vi "Graficas.vi"(1 "ID_EQUIPO":i32=1, 2 "Generador in":string) -> ()   [LabVIEW 2018]
uses:
  <vilib>/RAFA Solutions/Harmony UI Controls Kit/String & Path/String Indicator.ctl
  <vilib>/RAFA Solutions/Harmony UI Controls Kit/Boolean/OK Button.ctl
  <vilib>/addons/Electrical Power/Basic/Controls/Vector Diagram/EPX Vector Diagram.xctl
  Controls/Cluster_Potencias.ctl
  <vilib>/RAFA Solutions/Harmony UI Controls Kit/Numeric/Horizontal Progress Bar.ctl
  <vilib>/RAFA Solutions/Harmony UI Controls Kit/Boolean/Radio Button.ctl
  <vilib>/RAFA Solutions/Harmony UI Controls Kit/Boolean/Round Led.ctl
  Controls/Hora y Fecha control.ctl
  <vilib>/RAFA Solutions/Harmony UI Controls Kit/Boolean/Blank Button - Blue.ctl
  <vilib>/addons/database/Connection.llb/DB Tools Open Connec (Path).vi
  Global/Demo.vi
  Global/globalEventos.vi
  Global/Alarmas_indicadores-LED.vi
  <vilib>/RAFA Solutions/Harmony UI Controls Kit/Flat UI Design.lvlib
  <vilib>/addons/database/NI_Database_API.lvlib
panel:
  in  "type specifier VI Refnum (for type only) 2":refnum<vi>
  in  "ok":T1
  out "fecha y hora":T2
  out "Tol_Frec":T3 caption="TOL: Frecuencia"
  out "Mod_Frec":T3 caption="MOD: Frecuencia"
  out "Tol_V3_V1":T3 caption="TOL: V3_V1"
  out "Tol_V2_V3":T3 caption="TOL: V2_V3"
  out "Tol_V1_V2":T3 caption="TOL: V1_V2"
  out "Mod_V3_V1":T3 caption="MOD: V3_V1"
  out "Mod_V2_V3":T3 caption="MOD: V2_V3"
  out "Mod_V1_V2":T3 caption="MOD: V1_V2"
  out "G1_TRANS":T3 caption="Transiente"
  out "G1_SWELL":T3 caption="Swell"
  out "G1_SAG":T3 caption="Sag"
  in  "Seleccion Armonicos":T4(radio)
  out "Armónicos":sgl[](graph)
  out "?":sgl format="%#_3f"
  out "?":sgl format="%#_2f"
  out "?":sgl format="%#.1f"
  out "PROM":T5 scale=0.0..100.0
  out "L3-L1":T5 scale=0.0..100.0
  out "L2-L3":T5 scale=0.0..100.0
  out "L1-L2":T5 scale=0.0..100.0
  out "PROM.":T5 scale=0.0..100.0
  out "L3-L1":T5 scale=0.0..100.0
  out "L2-L3":T5 scale=0.0..100.0
  out "L1-L2":T5 scale=0.0..100.0
  out "TOTAL":T6 {"FACT. POT." scale=0.0..1.0; "APARENTE" scale=0.0..500.0; "REACTIVA" scale=0.0..500.0; "ACTIVA" scale=0.0..700.0}
  out "V3_V1":T6 {"FACT. POT." scale=0.0..1.0; "APARENTE" scale=0.0..500.0; "REACTIVA" scale=0.0..500.0; "ACTIVA" scale=0.0..700.0}
  out "V2-V3":T6 {"FACT. POT." scale=0.0..1.0; "APARENTE" scale=0.0..500.0; "REACTIVA" scale=0.0..500.0; "ACTIVA" scale=0.0..700.0}
  out "V1-V2":T6 {"FACT. POT." scale=0.0..1.0; "APARENTE" scale=0.0..500.0; "REACTIVA" scale=0.0..500.0; "ACTIVA" scale=0.0..700.0}
  out "Generador":string
  out "Corriente Vector Diagram":cdb[](xcontrol)
  out "Voltage Vector Diagram":cdb[](xcontrol)
  out "Frecuencia":cluster{"V1_V2":sgl, "V2_V3":sgl, "V3_V1":sgl}(graph)
  out "Corriente L_L":cluster{"V1_V2":sgl, "V2_V3":sgl, "V3_V1":sgl}(graph)
  out "Voltaje L-L":T7(graph)
  in  "volver":T8
  out "Eventos":T9
  # "Sistema de Monitoreo de Calidad de Energía"
  # "VOLTAJES L-L (RMS)"
  # "Gráfica Polar de Voltaje"
  # "POTENCIAS"
  # "VOLTAJE PROM."
  # "V"
  # "VALOR PROMEDIO \nV1-V2-V3"
  # "Límites de tolerancia según IEEE45"
  # "CORRIENTE PROM"
  # "A"
  # "VALOR PROMEDIO \nI1-I2-I3"
  # "CORRIENTES (RMS)"
  # "Gráfica Polar de Corriente"
  # "FRECUENCIA"
  # "Hz"
  # "THD VOLTAJE"
  # "THD CORRIENTE"
  # "%"
  # "%"
  # "ALARMAS"
  # "%"
  # "%"
  # "%"
  # "%"
  # "%"
  # "%"
  # "FRECUENCIA GENERADA"
  # "ARMÓNICOS"
  # "Límites de tolerancia según IEEE45"
  # "kW"
  # "kVAR"
  # "kVA"
  # "-"
  # "kW"
  # "kVAR"
  # "kVA"
  # "-"
  # "kW"
  # "kVAR"
  # "kVA"
  # "-"
  # "kW"
  # "kVAR"
  # "kVA"
  # "-"
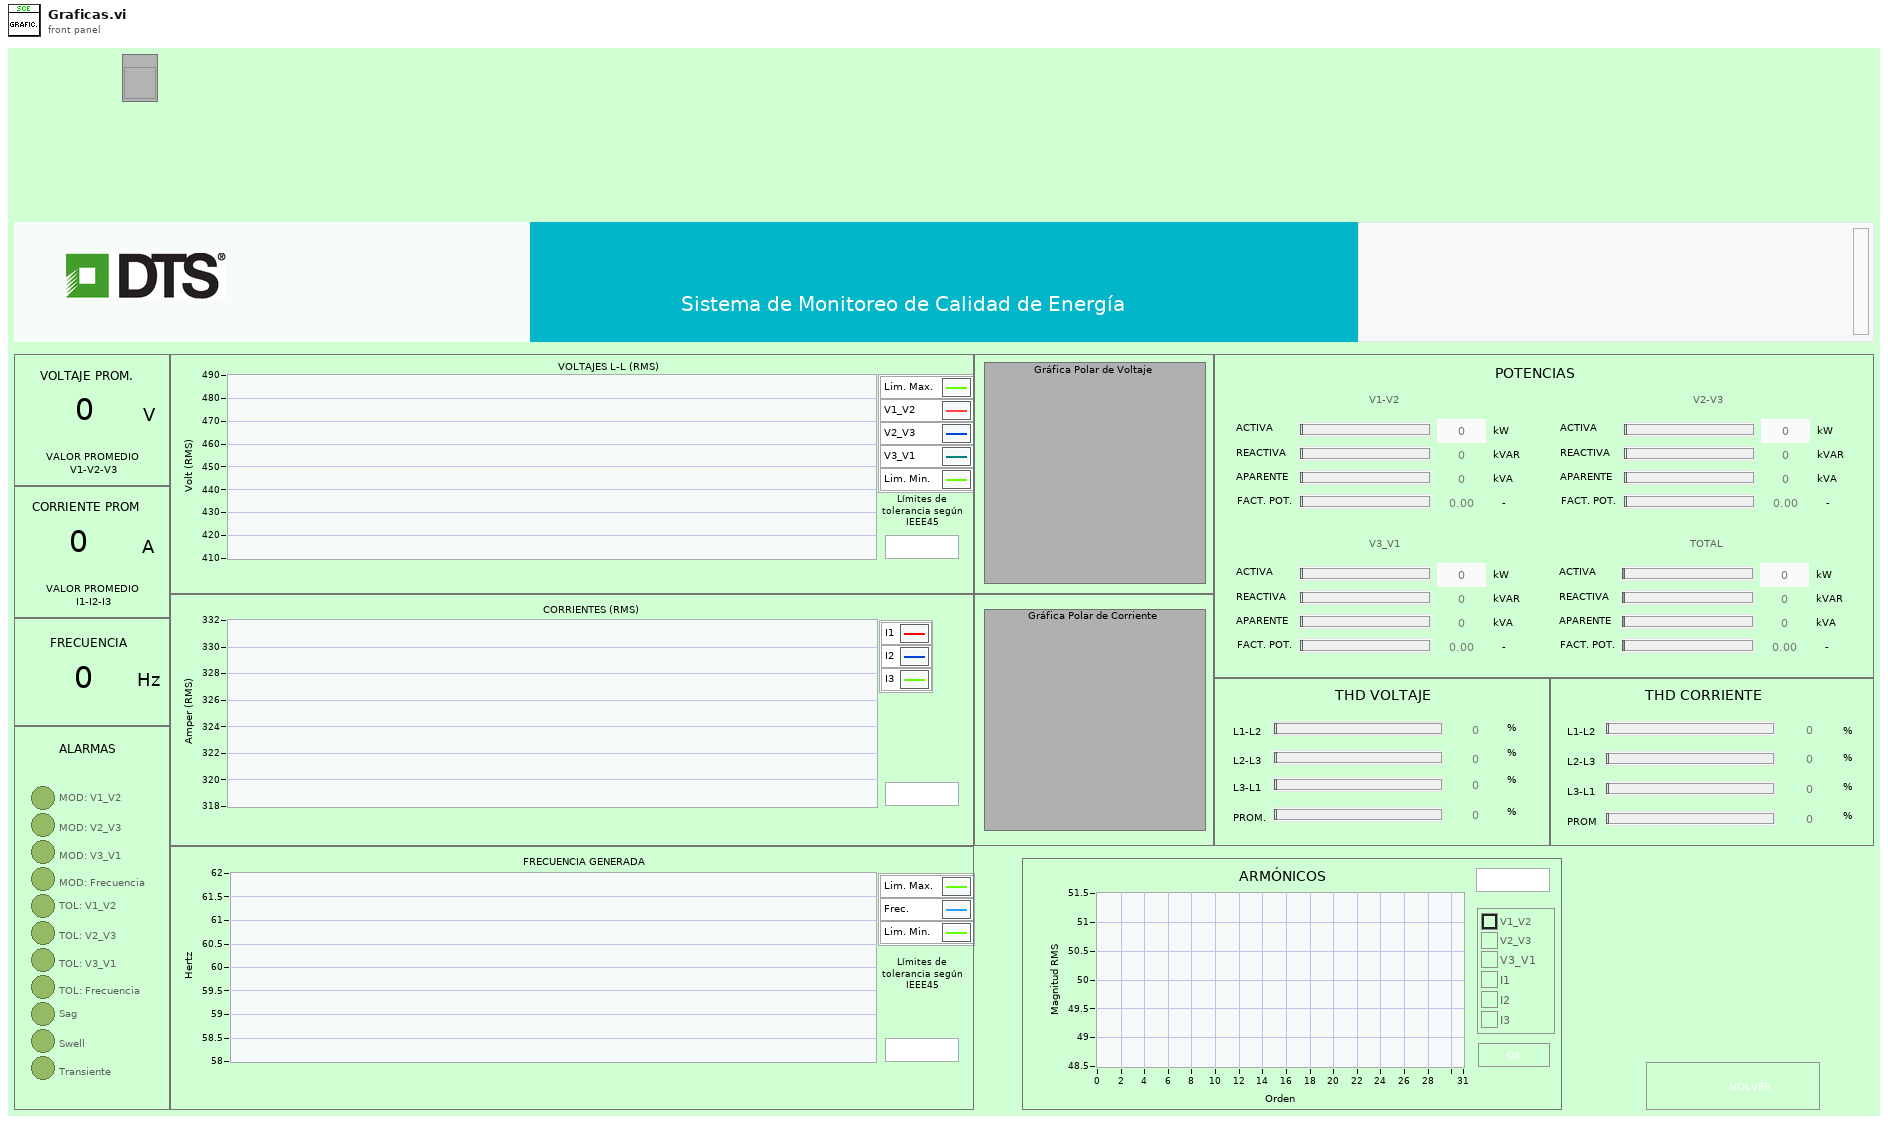
[diagram p1: front panel]
types:
  T1 = typedef "Flat UI Design.lvlib/Blank Button - Blue.ctl" = bool
  T2 = typedef "Hora y Fecha control.ctl" = cluster{"fecha":string, "dia semana":string, "fecha 2":string}
  T3 = typedef "Flat UI Design.lvlib/Round Led.ctl" = bool
  T4 = enum32{"V1_V2", "V2_V3", "V3_V1", "I1", "I2", "I3"}
  T5 = typedef "Flat UI Design.lvlib/Horizontal Progress Bar.ctl" = sgl
  T6 = typedef "Cluster_Potencias.ctl" = cluster{"ACTIVA":T5, "REACTIVA":T5, "APARENTE":T5, "FACT. POT.":T5}
  T7 = cluster{"Max":sgl, "V1_V2":sgl, "V2_V3":sgl, "V3_V1":sgl, "Min":sgl}
  T8 = typedef "Flat UI Design.lvlib/OK Button.ctl" = bool
  T9 = typedef "Flat UI Design.lvlib/String Indicator.ctl" = string
  T10 = cluster{"Max":sgl, "V1_V2":sgl, "V2_V3":sgl, "V3_V1":sgl, "Min":sgl}[]
  T11 = typedef "NI_Database_API.lvlib/Conn ObjectReference.ctl" = refnum<k1>
  T12 = cluster{"V_polar":cluster{"V1_ang":sgl, "V1_mag":sgl, "V2_ang":sgl, "V2_mag":sgl, "V3_ang":sgl, "V3_mag":sgl}, "I_polar":cluster{"I1_ang":sgl, "I1_mag":sgl, "I2_ang":sgl, "I2_mag":sgl, "I3_ang":sgl, "I3_mag":sgl}}
  T13 = typedef "THD_cluster.ctl" = cluster{"V_THD":cluster{"V1_V2_THD":sgl, "V2_V3_THD":sgl, "V3_V1_THD":sgl, "Avg_V_V_THD":sgl}, "I_THD":cluster{"I1_THD":sgl, "I2_THD":sgl, "I3_THD":sgl, "I4_THD":sgl, "Avg_I_THD":sgl}}
  T14 = cluster{"V1_V2_THD":sgl, "V2_V3_THD":sgl, "V3_V1_THD":sgl, "Avg_V_V_THD":sgl}
  T15 = cluster{"I1_THD":sgl, "I2_THD":sgl, "I3_THD":sgl, "I4_THD":sgl, "Avg_I_THD":sgl}
  T16 = cluster{"Real Power (kW)":cluster{"L1_kW":sgl, "L2_kW":sgl, "L3_kW":sgl, "Total_kW":sgl}, "Reactive Power (kVAR)":cluster{"L1_kVAR":sgl, "L2_kVAR":sgl, "L3_kVAR":sgl, "Total_kVAR":sgl}, "Aparent Power (kVA)":cluster{"L1_kVA":sgl, "L2_kVA":sgl, "L3_kVA":sgl, "Total_kVA":sgl}, "Power Factor":cluster{"L1_PF":sgl, "L2_PF":sgl, "L3_PF":sgl, "Total_PF":sgl}}
  T17 = cluster{"Real Power (kW)":cluster{"L1_kW":sgl, "L2_kW":sgl, "L3_kW":sgl, "Total_kW":sgl}, "Reactive Power (kVAR)":cluster{"L1_kVAR":sgl, "L2_kVAR":sgl, "L3_kVAR":sgl, "Total_kVAR":sgl}, "Aparent Power (kVA)":cluster{"L1_kVA":sgl, "L2_kVA":sgl, "L3_kVA":sgl, "Total_kVA":sgl}, "Power Factor (%)":cluster{"L1_PF":sgl, "L2_PF":sgl, "L3_PF":sgl, "Total_PF":sgl}}
  T18 = cluster{"L1_kW":sgl, "L2_kW":sgl, "L3_kW":sgl, "Total_kW":sgl}
  T19 = cluster{"L1_kVAR":sgl, "L2_kVAR":sgl, "L3_kVAR":sgl, "Total_kVAR":sgl}
  T20 = cluster{"L1_kVA":sgl, "L2_kVA":sgl, "L3_kVA":sgl, "Total_kVA":sgl}
  T21 = cluster{"L1_PF":sgl, "L2_PF":sgl, "L3_PF":sgl, "Total_PF":sgl}
  T22 = typedef "VIF_cluster.ctl" = cluster{"VL_VL":cluster{"V1_V2":sgl, "V2_V3":sgl, "V3_V1":sgl, "Avg_VL_VL":sgl}, "IL_IL":cluster{"I1":sgl, "I2":sgl, "I3":sgl, "Avg_Amps":sgl}, "Frecuency":sgl, "Avg_Frecuency":sgl}
  T23 = cluster{"V1_V2":sgl, "V2_V3":sgl, "V3_V1":sgl, "Avg_VL_VL":sgl}
  T24 = cluster{"I1":sgl, "I2":sgl, "I3":sgl, "Avg_Amps":sgl}
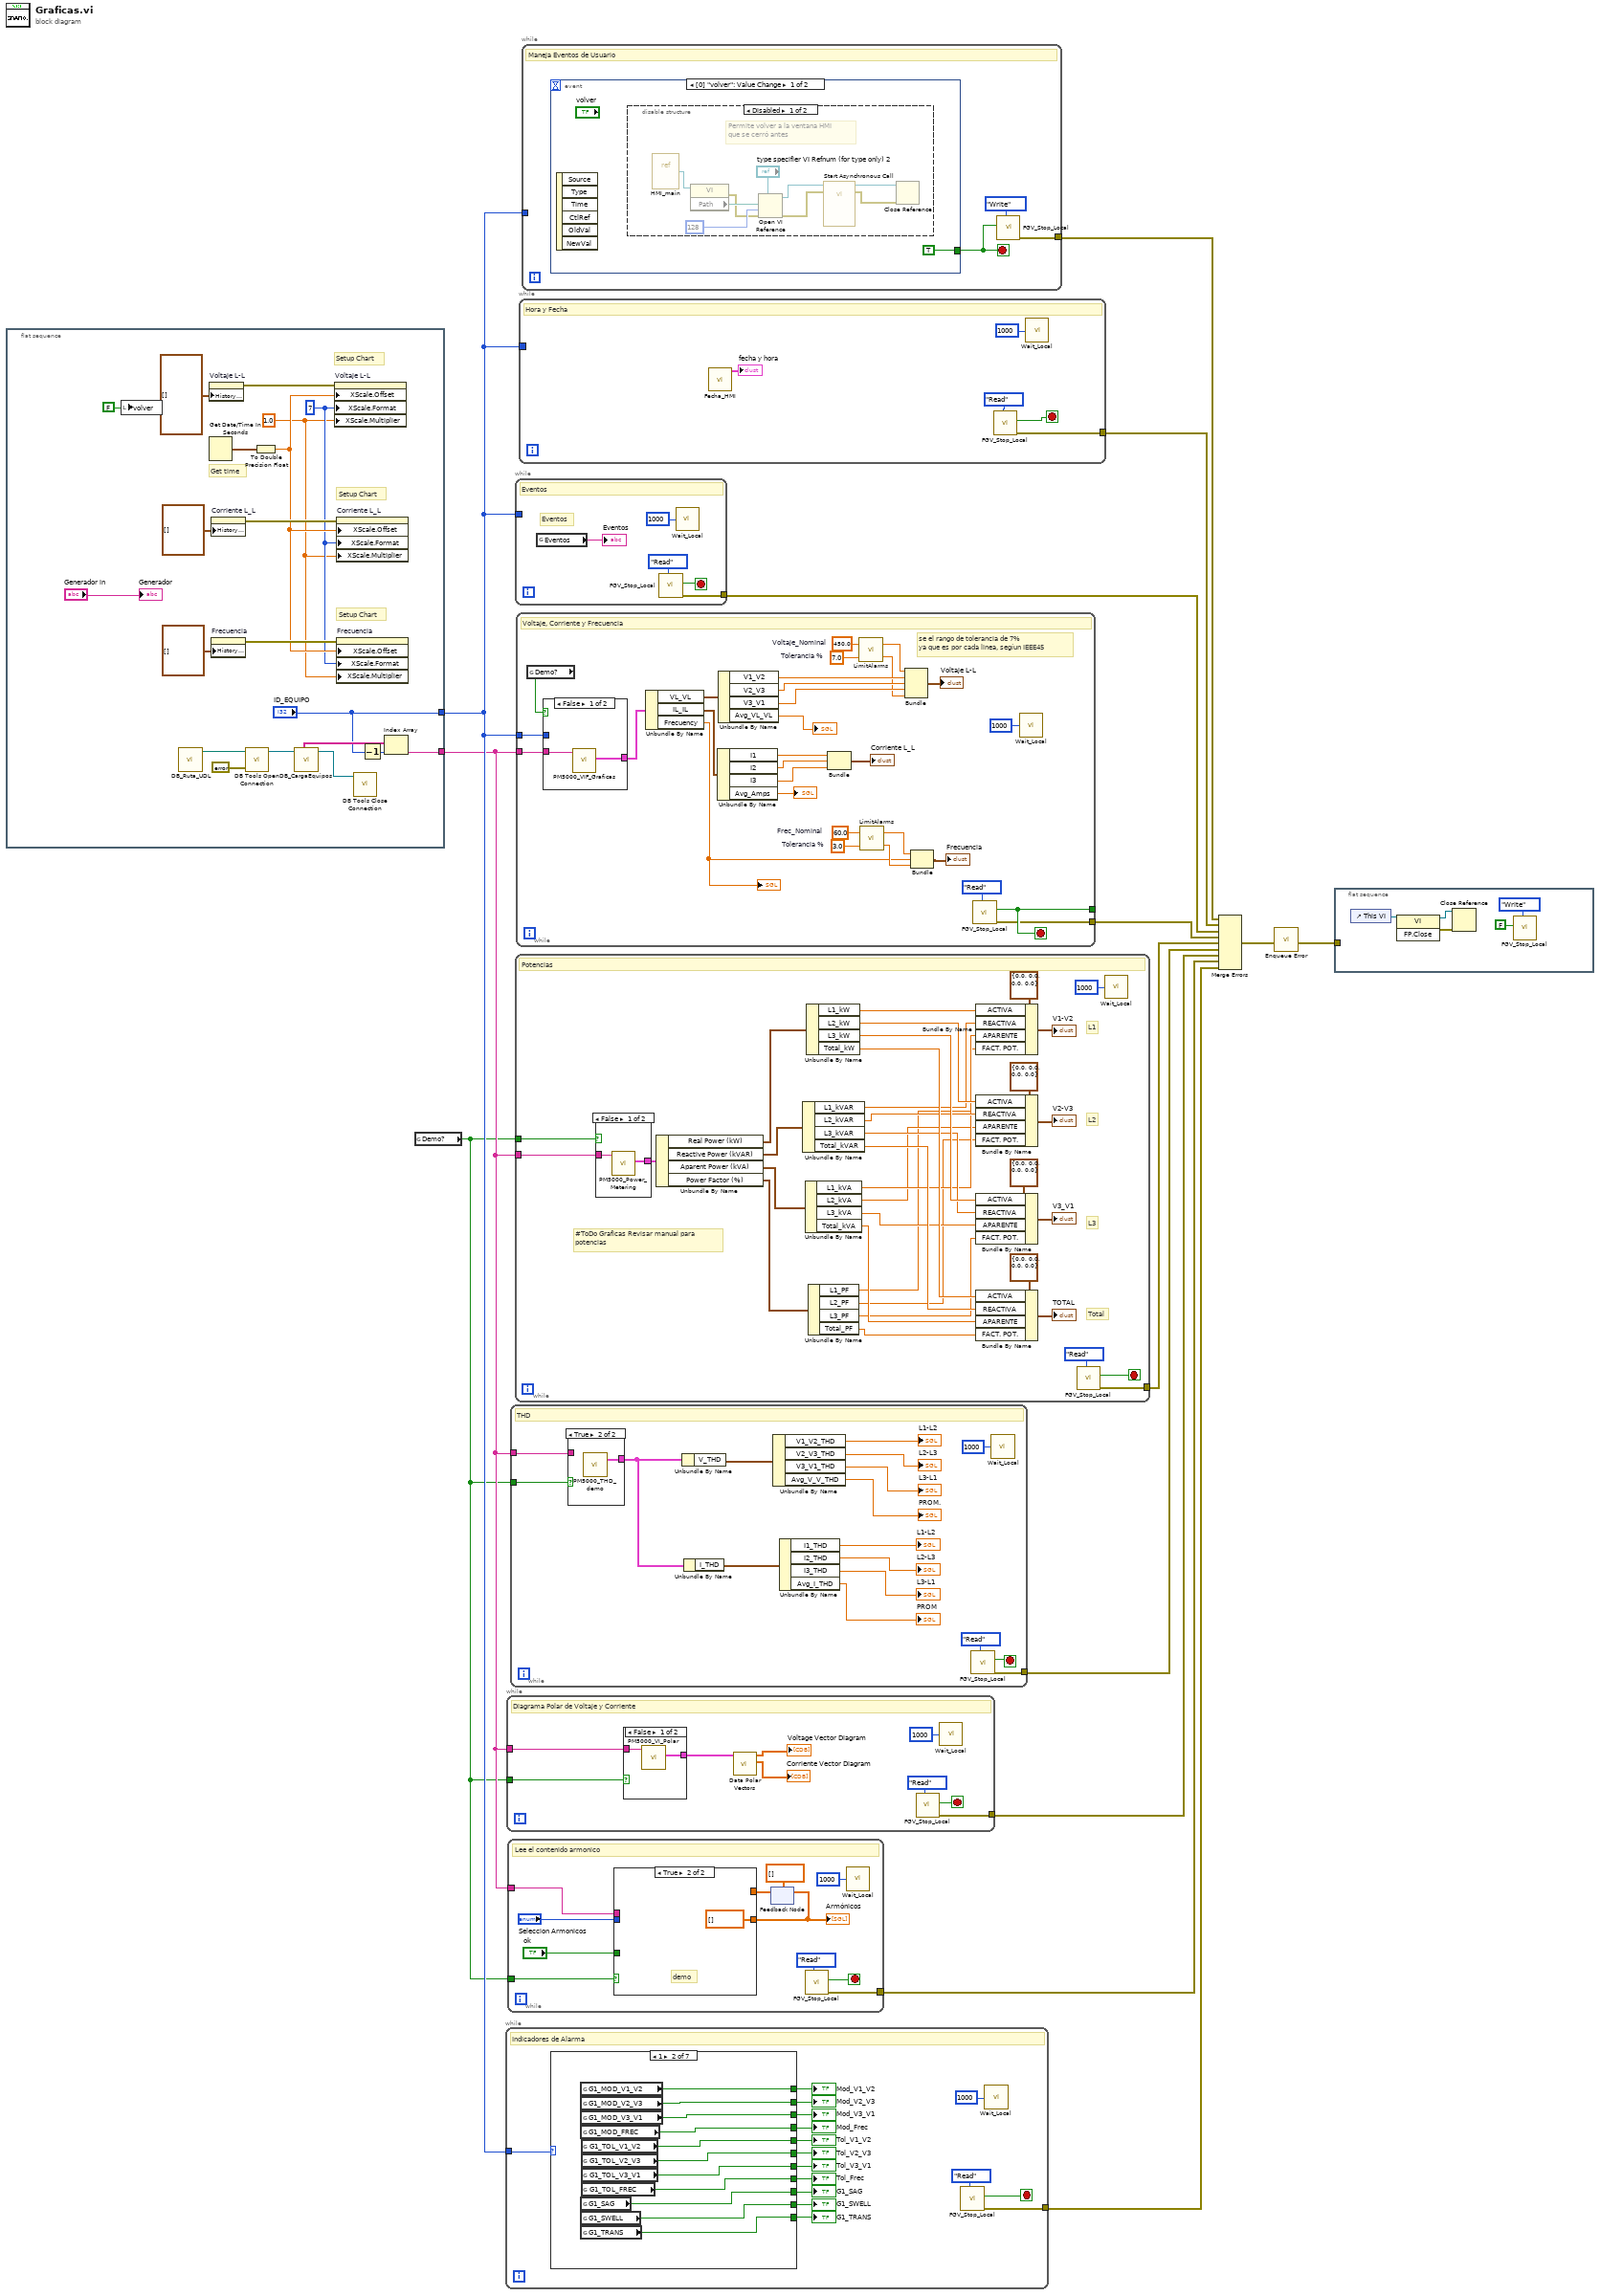
[diagram p0: block diagram]
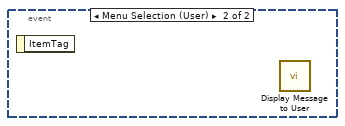
[diagram p3: hidden frame]
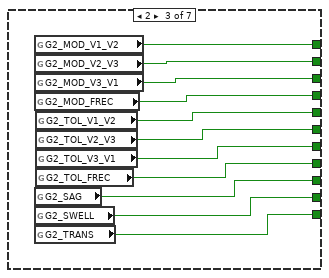
[diagram p5: hidden frame]
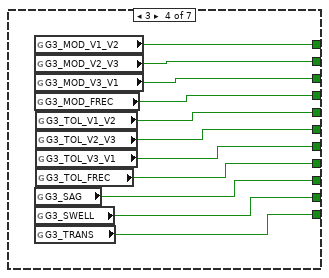
[diagram p6: hidden frame]
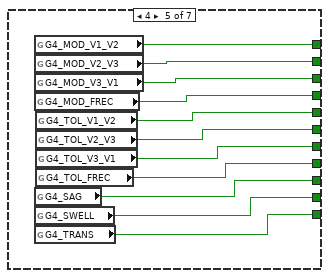
[diagram p7: hidden frame]
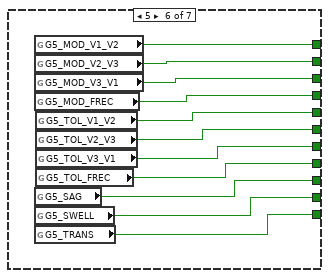
[diagram p8: hidden frame]
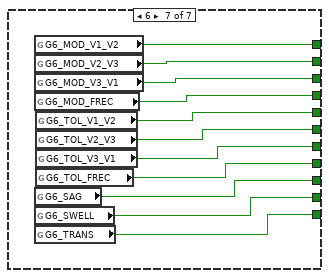
[diagram p9: hidden frame]
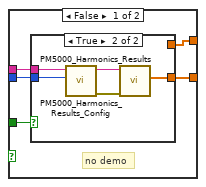
[diagram p10: hidden frame]
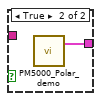
[diagram p12: hidden frame]
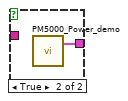
[diagram p13: hidden frame]
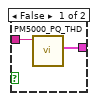
[diagram p14: hidden frame]
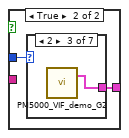
[diagram p15: hidden frame]
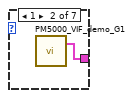
[diagram p17: hidden frame]
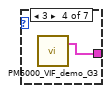
[diagram p18: hidden frame]
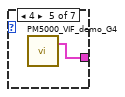
[diagram p19: hidden frame]
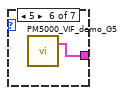
[diagram p20: hidden frame]
diagram:
  n1 = flat-sequence {
    tunnel: ["ID_EQUIPO"] -> w3
    tunnel: [w16] -> w2
    frame #0 {
      w23 = 1.0 ("X Scale.Offset and Multiplier:Multiplier")
      w25 = u8 7 ("X Scale.Display Format:Format")
      # "Setup Chart"
      # "Setup Chart"
      # "Get time"
      # "Setup Chart"
      n2 = local write "volver"(T8 FALSE ("volver")) -> ()
      n3 = call "DB_Ruta_UDL.vi"() -> ("UDL ruta"=w18:path)  [unwired: 11 in]
      n4 = property on="Voltaje L-L" class="WFChart (strict)"("History Data"=T10 []) -> (error out=w33:errorcluster)  [unwired: 2 in, 1 out]
      n5 = Get Date/Time In Seconds() -> (seconds since 1Jan1904=w34:timestamp)
      n6 = property on="Corriente L_L" class="WFChart (strict)"("History Data"=cluster{"V1_V2":sgl, "V2_V3":sgl, "V3_V1":sgl}[] []) -> (error out=w32:errorcluster)  [unwired: 2 in, 1 out]
      n7 = property on="Frecuencia" class="WFChart (strict)"("History Data"=cluster{"V1_V2":sgl, "V2_V3":sgl, "V3_V1":sgl}[] []) -> (error out=w31:errorcluster)  [unwired: 2 in, 1 out]
      n8 = call-poly <vilib>:"DB Tools Open Connection.vi"("error in (no error)"=errorcluster {"status"=FALSE, "code"=0, "source"=""}, "connection information"=w18) -> ("connection reference"=w19:T11)  [unwired: 6 in, 1 out]
      n9 = To Double Precision Float(number=w34) -> (double precision float=w30:dbl)
      n10 = call "DB_CargaEquipos.vi"("db in"=w19) -> ("db out"=w15:T11, "IP_EQUIPOS"=w21:string[])  [unwired: 3 in, 6 out]
      n11 = property on="Voltaje L-L" class="WFChart (strict)"(error in=w33, "XScale.Offset"=w30, "XScale.Format"=w25, "XScale.Multiplier"=w23) -> ()  [unwired: 1 in, 2 out]
      n12 = property on="Corriente L_L" class="WFChart (strict)"(error in=w32, "XScale.Offset"=w30, "XScale.Format"=w25, "XScale.Multiplier"=w23) -> ()  [unwired: 1 in, 2 out]
      n13 = property on="Frecuencia" class="WFChart (strict)"(error in=w31, "XScale.Offset"=w30, "XScale.Format"=w25, "XScale.Multiplier"=w23) -> ()  [unwired: 1 in, 2 out]
      n14 = call <vilib>:"DB Tools Close Connection.vi"("connection reference"=w15) -> ()  [unwired: 6 in, 1 out]
      n15 = Decrement(x="ID_EQUIPO") -> (x-1=w20:i32)
      n16 = Index Array(array=w21, index=w20) -> (element=w16:string)
      "Generador" <- "Generador in"
    }
  }
  n17 = global read "Demo.vi" "Demo?"() -> (w1:bool)
  n18 = while {
    tunnel: [w47] -> w6
    tunnel: w3 -> [w35]
    stop <- w48 stop-if-true
    # "Indicadores de Alarma"
    n19 = case shown="1" w35 {
      tunnel: [_ w61 w72 w83 w94 w105 w116] -> w46
      tunnel: [_ w60 w71 w82 w93 w104 w115] -> w45
      tunnel: [_ w59 w70 w81 w92 w103 w114] -> w44
      tunnel: [_ w58 w69 w80 w91 w102 w113] -> w43
      tunnel: [_ w57 w68 w79 w90 w101 w112] -> w42
      tunnel: [_ w56 w67 w78 w89 w100 w111] -> w41
      tunnel: [_ w55 w66 w77 w88 w99 w110] -> w40
      tunnel: [_ w54 w65 w76 w87 w98 w109] -> w39
      tunnel: [_ w53 w64 w75 w86 w97 w108] -> w38
      tunnel: [_ w52 w63 w74 w85 w96 w107] -> w37
      tunnel: [_ w51 w62 w73 w84 w95 w106] -> w36
      frame 0, Default {
      }
      frame 1 {
        n20 = global read "Alarmas_indicadores-LED.vi" "G1_MOD_V1_V2"() -> (w61:bool)
        n21 = global read "Alarmas_indicadores-LED.vi" "G1_MOD_V2_V3"() -> (w60:bool)
        n22 = global read "Alarmas_indicadores-LED.vi" "G1_MOD_V3_V1"() -> (w59:bool)
        n23 = global read "Alarmas_indicadores-LED.vi" "G1_MOD_FREC"() -> (w58:bool)
        n24 = global read "Alarmas_indicadores-LED.vi" "G1_SAG"() -> (w53:bool)
        n25 = global read "Alarmas_indicadores-LED.vi" "G1_SWELL"() -> (w52:bool)
        n26 = global read "Alarmas_indicadores-LED.vi" "G1_TRANS"() -> (w51:bool)
        n27 = global read "Alarmas_indicadores-LED.vi" "G1_TOL_V1_V2"() -> (w57:bool)
        n28 = global read "Alarmas_indicadores-LED.vi" "G1_TOL_V2_V3"() -> (w56:bool)
        n29 = global read "Alarmas_indicadores-LED.vi" "G1_TOL_V3_V1"() -> (w55:bool)
        n30 = global read "Alarmas_indicadores-LED.vi" "G1_TOL_FREC"() -> (w54:bool)
      }
      frame 2 {
        n31 = global read "Alarmas_indicadores-LED.vi" "G2_MOD_V1_V2"() -> (w72:bool)
        n32 = global read "Alarmas_indicadores-LED.vi" "G2_MOD_V2_V3"() -> (w71:bool)
        n33 = global read "Alarmas_indicadores-LED.vi" "G2_MOD_V3_V1"() -> (w70:bool)
        n34 = global read "Alarmas_indicadores-LED.vi" "G2_MOD_FREC"() -> (w69:bool)
        n35 = global read "Alarmas_indicadores-LED.vi" "G2_SAG"() -> (w64:bool)
        n36 = global read "Alarmas_indicadores-LED.vi" "G2_SWELL"() -> (w63:bool)
        n37 = global read "Alarmas_indicadores-LED.vi" "G2_TRANS"() -> (w62:bool)
        n38 = global read "Alarmas_indicadores-LED.vi" "G2_TOL_V1_V2"() -> (w68:bool)
        n39 = global read "Alarmas_indicadores-LED.vi" "G2_TOL_V2_V3"() -> (w67:bool)
        n40 = global read "Alarmas_indicadores-LED.vi" "G2_TOL_V3_V1"() -> (w66:bool)
        n41 = global read "Alarmas_indicadores-LED.vi" "G2_TOL_FREC"() -> (w65:bool)
      }
      frame 3 {
        n42 = global read "Alarmas_indicadores-LED.vi" "G3_MOD_V1_V2"() -> (w83:bool)
        n43 = global read "Alarmas_indicadores-LED.vi" "G3_MOD_V2_V3"() -> (w82:bool)
        n44 = global read "Alarmas_indicadores-LED.vi" "G3_MOD_V3_V1"() -> (w81:bool)
        n45 = global read "Alarmas_indicadores-LED.vi" "G3_MOD_FREC"() -> (w80:bool)
        n46 = global read "Alarmas_indicadores-LED.vi" "G3_SAG"() -> (w75:bool)
        n47 = global read "Alarmas_indicadores-LED.vi" "G3_SWELL"() -> (w74:bool)
        n48 = global read "Alarmas_indicadores-LED.vi" "G3_TRANS"() -> (w73:bool)
        n49 = global read "Alarmas_indicadores-LED.vi" "G3_TOL_V1_V2"() -> (w79:bool)
        n50 = global read "Alarmas_indicadores-LED.vi" "G3_TOL_V2_V3"() -> (w78:bool)
        n51 = global read "Alarmas_indicadores-LED.vi" "G3_TOL_V3_V1"() -> (w77:bool)
        n52 = global read "Alarmas_indicadores-LED.vi" "G3_TOL_FREC"() -> (w76:bool)
      }
      frame 4 {
        n53 = global read "Alarmas_indicadores-LED.vi" "G4_MOD_V1_V2"() -> (w94:bool)
        n54 = global read "Alarmas_indicadores-LED.vi" "G4_MOD_V2_V3"() -> (w93:bool)
        n55 = global read "Alarmas_indicadores-LED.vi" "G4_MOD_V3_V1"() -> (w92:bool)
        n56 = global read "Alarmas_indicadores-LED.vi" "G4_MOD_FREC"() -> (w91:bool)
        n57 = global read "Alarmas_indicadores-LED.vi" "G4_SAG"() -> (w86:bool)
        n58 = global read "Alarmas_indicadores-LED.vi" "G4_SWELL"() -> (w85:bool)
        n59 = global read "Alarmas_indicadores-LED.vi" "G4_TRANS"() -> (w84:bool)
        n60 = global read "Alarmas_indicadores-LED.vi" "G4_TOL_V1_V2"() -> (w90:bool)
        n61 = global read "Alarmas_indicadores-LED.vi" "G4_TOL_V2_V3"() -> (w89:bool)
        n62 = global read "Alarmas_indicadores-LED.vi" "G4_TOL_V3_V1"() -> (w88:bool)
        n63 = global read "Alarmas_indicadores-LED.vi" "G4_TOL_FREC"() -> (w87:bool)
      }
      frame 5 {
        n64 = global read "Alarmas_indicadores-LED.vi" "G5_MOD_V1_V2"() -> (w105:bool)
        n65 = global read "Alarmas_indicadores-LED.vi" "G5_MOD_V2_V3"() -> (w104:bool)
        n66 = global read "Alarmas_indicadores-LED.vi" "G5_MOD_V3_V1"() -> (w103:bool)
        n67 = global read "Alarmas_indicadores-LED.vi" "G5_MOD_FREC"() -> (w102:bool)
        n68 = global read "Alarmas_indicadores-LED.vi" "G5_SAG"() -> (w97:bool)
        n69 = global read "Alarmas_indicadores-LED.vi" "G5_SWELL"() -> (w96:bool)
        n70 = global read "Alarmas_indicadores-LED.vi" "G5_TRANS"() -> (w95:bool)
        n71 = global read "Alarmas_indicadores-LED.vi" "G5_TOL_V1_V2"() -> (w101:bool)
        n72 = global read "Alarmas_indicadores-LED.vi" "G5_TOL_V2_V3"() -> (w100:bool)
        n73 = global read "Alarmas_indicadores-LED.vi" "G5_TOL_V3_V1"() -> (w99:bool)
        n74 = global read "Alarmas_indicadores-LED.vi" "G5_TOL_FREC"() -> (w98:bool)
      }
      frame 6 {
        n75 = global read "Alarmas_indicadores-LED.vi" "G6_MOD_V1_V2"() -> (w116:bool)
        n76 = global read "Alarmas_indicadores-LED.vi" "G6_MOD_V2_V3"() -> (w115:bool)
        n77 = global read "Alarmas_indicadores-LED.vi" "G6_MOD_V3_V1"() -> (w114:bool)
        n78 = global read "Alarmas_indicadores-LED.vi" "G6_MOD_FREC"() -> (w113:bool)
        n79 = global read "Alarmas_indicadores-LED.vi" "G6_SAG"() -> (w108:bool)
        n80 = global read "Alarmas_indicadores-LED.vi" "G6_SWELL"() -> (w107:bool)
        n81 = global read "Alarmas_indicadores-LED.vi" "G6_TRANS"() -> (w106:bool)
        n82 = global read "Alarmas_indicadores-LED.vi" "G6_TOL_V1_V2"() -> (w112:bool)
        n83 = global read "Alarmas_indicadores-LED.vi" "G6_TOL_V2_V3"() -> (w111:bool)
        n84 = global read "Alarmas_indicadores-LED.vi" "G6_TOL_V3_V1"() -> (w110:bool)
        n85 = global read "Alarmas_indicadores-LED.vi" "G6_TOL_FREC"() -> (w109:bool)
      }
    }
    "Mod_V1_V2" <- w46
    "Mod_V2_V3" <- w45
    "Mod_V3_V1" <- w44
    "Mod_Frec" <- w43
    "Tol_V1_V2" <- w42
    "Tol_V2_V3" <- w41
    "Tol_V3_V1" <- w40
    "Tol_Frec" <- w39
    "G1_SAG" <- w38
    "G1_SWELL" <- w37
    "G1_TRANS" <- w36
    n86 = call "FGV_Stop_Local.vi"("Action"=enum16{"Read", "Write"}."Read") -> ("Error Out"=w47:errorcluster, "Var Out"=w48:bool)  [unwired: 9 in]
    n87 = call "Wait_Local.vi"("Wait time (msec)"=u32 1000 ("milliseconds to wait")) -> ()  [unwired: 5 in]
  }
  n88 = while {
    tunnel: [w119] -> w9
    tunnel: w1 -> [w118]
    tunnel: w2 -> [w117]
    stop <- w124 stop-if-true
    # "Diagrama Polar de Voltaje y Corriente"
    n89 = case shown="False" w118 {
      tunnel: [w127 w128] -> w123
      tunnel: w117 -> [w126 _]
      frame False {
        n90 = call "PM5000_VI_Polar.vi"("Network Path"=w126) -> ("VI_polar out"=w127:T12)  [unwired: 7 in, 3 out]
      }
      frame True {
        n91 = call "PM5000_Polar_demo.vi"() -> ("VI_polar out"=w128:T12)  [unwired: 2 in, 1 out]
      }
    }
    n92 = call "Data Polar Vectors.vi"("Polar_VI"=w123) -> ("current vectors"=→"Corriente Vector Diagram":cdb[], "voltage vectors"=→"Voltage Vector Diagram":cdb[])  [unwired: 8 in, 1 out]
    n93 = call "FGV_Stop_Local.vi"("Action"=enum16{"Read", "Write"}."Read") -> ("Error Out"=w119:errorcluster, "Var Out"=w124:bool)  [unwired: 9 in]
    n94 = call "Wait_Local.vi"("Wait time (msec)"=u32 1000 ("milliseconds to wait")) -> ()  [unwired: 5 in]
  }
  n95 = while {
    tunnel: w2 -> [w137]
    tunnel: [w135] -> w8
    tunnel: w1 -> [w130]
    stop <- w138 stop-if-true
    # "Lee el contenido armonico"
    n96 = feedback #1(sgl[] [] ("harmonics out")) -> (w132:sgl[])
    n97 = case shown="True" w130 {
      tunnel: w137 -> [w144 _]
      tunnel: "Seleccion Armonicos" -> [w143 _]
      tunnel: "ok" -> [w142 _]
      tunnel: [w141 sgl[] [] ("harmonics out")] -> w133
      tunnel: w132 -> [w140 _]
      frame False {
        # "no demo"
        n98 = case shown="True" w142 {
          tunnel: w144 -> [_ w150]
          tunnel: [w145 w149] -> w141
          tunnel: w143 -> [_ w148]
          tunnel: w140 -> [w145 _]
          frame False {
          }
          frame True {
            n99 = call "PM5000_Harmonics_Results_Config.vi"("Seleccion Armonicos"=w148, "Network Path"=w150) -> ("error out"=w146:errorcluster, "Network Path out"=w147:string)  [unwired: 8 in]
            n100 = call "PM5000_Harmonics_Results.vi"("error in"=w146, "Network Path"=w147) -> ("harmonics out"=w149:sgl[])  [unwired: 7 in, 2 out]
          }
        }
      }
      frame True {
        # "demo"
      }
    }
    "Armónicos" <- w133
    n101 = feedback-in #1(w133) -> ()
    n102 = call "FGV_Stop_Local.vi"("Action"=enum16{"Read", "Write"}."Read") -> ("Error Out"=w135:errorcluster, "Var Out"=w138:bool)  [unwired: 9 in]
    n103 = call "Wait_Local.vi"("Wait time (msec)"=u32 1000 ("milliseconds to wait")) -> ()  [unwired: 5 in]
  }
  n104 = while {
    tunnel: [w154] -> w10
    tunnel: w1 -> [w153]
    tunnel: w2 -> [w152]
    stop <- w158 stop-if-true
    # "THD"
    n105 = case shown="True" w153 {
      tunnel: [w169 w171] -> w156
      tunnel: w152 -> [w170 _]
      frame False {
        n106 = call "PM5000_PQ_THD.vi"("Network Path"=w170) -> ("THD_cluster"=w169:T13)  [unwired: 7 in, 3 out]
      }
      frame True {
        n107 = call "PM5000_THD_demo.vi"() -> ("THD_cluster"=w171:T13)  [unwired: 2 in, 1 out]
      }
    }
    n108 = Unbundle By Name(w156) -> ("V_THD"=w168:T14)
    n109 = Unbundle By Name(w156) -> ("I_THD"=w167:T15)
    n110 = Unbundle By Name(w168) -> ("V1_V2_THD"=→"L1-L2":sgl, "V2_V3_THD"=→"L2-L3":sgl, "V3_V1_THD"=→"L3-L1":sgl, "Avg_V_V_THD"=→"PROM.":sgl)
    n111 = Unbundle By Name(w167) -> ("I1_THD"=→"L1-L2":sgl, "I2_THD"=→"L2-L3":sgl, "I3_THD"=→"L3-L1":sgl, "Avg_I_THD"=→"PROM":sgl)
    n112 = call "FGV_Stop_Local.vi"("Action"=enum16{"Read", "Write"}."Read") -> ("Error Out"=w154:errorcluster, "Var Out"=w158:bool)  [unwired: 9 in]
    n113 = call "Wait_Local.vi"("Wait time (msec)"=u32 1000 ("milliseconds to wait")) -> ()  [unwired: 5 in]
  }
  n114 = while {
    tunnel: [w174] -> w11
    tunnel: w1 -> [w173]
    tunnel: w2 -> [w172]
    stop <- w175 stop-if-true
    # "#ToDo Graficas Revisar manual para \npotencias"
    # "Total"
    # "L3"
    # "L2"
    # "L1"
    # "Potencias"
    n115 = case shown="False" w173 {
      tunnel: [w208 w209] -> w206
      tunnel: w172 -> [w207 _]
      frame False {
        n116 = call "PM5000_Power_Metering.vi"("Network Path"=w207) -> ("Power Meter Out"=w208:T16)  [unwired: 7 in, 3 out]
      }
      frame True {
        n117 = call "PM5000_Power_demo.vi"() -> ("Power Meter Out"=w209:T17)  [unwired: 2 in, 1 out]
      }
    }
    n118 = Unbundle By Name(w206) -> ("Real Power (kW)"=w197:T18, "Reactive Power (kVAR)"=w196:T19, "Aparent Power (kVA)"=w195:T20, "Power Factor (%)"=w194:T21)
    n119 = Unbundle By Name(w196) -> ("L1_kVAR"=w189:sgl, "L2_kVAR"=w188:sgl, "L3_kVAR"=w187:sgl, "Total_kVAR"=w186:sgl)
    n120 = Unbundle By Name(w195) -> ("L1_kVA"=w185:sgl, "L2_kVA"=w184:sgl, "L3_kVA"=w183:sgl, "Total_kVA"=w182:sgl)
    n121 = Unbundle By Name(w197) -> ("L1_kW"=w193:sgl, "L2_kW"=w192:sgl, "L3_kW"=w191:sgl, "Total_kW"=w190:sgl)
    n122 = Unbundle By Name(w194) -> ("L1_PF"=w181:sgl, "L2_PF"=w180:sgl, "L3_PF"=w179:sgl, "Total_PF"=w178:sgl)
    n123 = Bundle By Name(cluster=T6 {"ACTIVA"=0.0, "REACTIVA"=0.0, "APARENTE"=0.0, "FACT. POT."=0.0} ("V1-V2"), "ACTIVA"=w193, "REACTIVA"=w189, "APARENTE"=w185, "FACT. POT."=w181) -> (→"V1-V2":T6)
    n124 = Bundle By Name(cluster=T6 {"ACTIVA"=0.0, "REACTIVA"=0.0, "APARENTE"=0.0, "FACT. POT."=0.0} ("V2-V3"), "ACTIVA"=w192, "REACTIVA"=w188, "APARENTE"=w184, "FACT. POT."=w180) -> (→"V2-V3":T6)
    n125 = Bundle By Name(cluster=T6 {"ACTIVA"=0.0, "REACTIVA"=0.0, "APARENTE"=0.0, "FACT. POT."=0.0} ("V3_V1"), "ACTIVA"=w191, "REACTIVA"=w187, "APARENTE"=w183, "FACT. POT."=w179) -> (→"V3_V1":T6)
    n126 = Bundle By Name(cluster=T6 {"ACTIVA"=0.0, "REACTIVA"=0.0, "APARENTE"=0.0, "FACT. POT."=0.0} ("TOTAL"), "ACTIVA"=w190, "REACTIVA"=w186, "APARENTE"=w182, "FACT. POT."=w178) -> (→"TOTAL":T6)
    n127 = call "FGV_Stop_Local.vi"("Action"=enum16{"Read", "Write"}."Read") -> ("Error Out"=w174:errorcluster, "Var Out"=w175:bool)  [unwired: 9 in]
    n128 = call "Wait_Local.vi"("Wait time (msec)"=u32 1000 ("milliseconds to wait")) -> ()  [unwired: 5 in]
  }
  n129 = while {
    tunnel: [w211] -> w13
    tunnel: w3 -> [_]
    stop <- w213 stop-if-true
    # "Eventos"
    # "Eventos"
    n130 = global read "globalEventos.vi" "Eventos"() -> (→"Eventos":string)
    n131 = call "FGV_Stop_Local.vi"("Action"=enum16{"Read", "Write"}."Read") -> ("Error Out"=w211:errorcluster, "Var Out"=w213:bool)  [unwired: 9 in]
    n132 = call "Wait_Local.vi"("Wait time (msec)"=u32 1000 ("milliseconds to wait")) -> ()  [unwired: 5 in]
  }
  n133 = while {
    tunnel: [w221] -> _
    tunnel: [w219] -> w12
    tunnel: w2 -> [w218]
    tunnel: w3 -> [w215]
    stop <- w221 stop-if-true
    w227 = sgl 3.0  # Tolerancia %
    w226 = sgl 60.0  # Frec_Nominal
    w239 = sgl 7.0  # Tolerancia %
    w240 = sgl 450.0  # Voltaje_Nominal
    # "se el rango de tolerancia de 7%\nya que es por cada linea, segíun IEEE45"
    # "Voltaje, Corriente y Frecuencia"
    n134 = global read "Demo.vi" "Demo?"() -> (w216:bool)
    n135 = case shown="False" w216 {
      tunnel: w218 -> [w246 _]
      tunnel: [w245 w247] -> w217
      tunnel: w215 -> [_ w248]
      frame False {
        n136 = call "PM5000_VIF_Graficas.vi"("Network Path"=w246) -> ("output cluster"=w245:T22)  [unwired: 8 in, 2 out]
      }
      frame True {
        n137 = case shown="2" w248 {
          tunnel: [_ w249 w250 w251 w252 w253 w254] -> w247
          frame Default {
          }
          frame 1 {
            n138 = call "PM5000_VIF_demo_G1.vi"() -> ("VIF_cluster"=w249:T22)  [unwired: 2 in, 1 out]
          }
          frame 2 {
            n139 = call "PM5000_VIF_demo_G2.vi"() -> ("VIF_cluster"=w250:T22)  [unwired: 2 in, 1 out]
          }
          frame 3 {
            n140 = call "PM5000_VIF_demo_G3.vi"() -> ("VIF_cluster"=w251:T22)  [unwired: 2 in, 1 out]
          }
          frame 4 {
            n141 = call "PM5000_VIF_demo_G4.vi"() -> ("VIF_cluster"=w252:T22)  [unwired: 2 in, 1 out]
          }
          frame 5 {
            n142 = call "PM5000_VIF_demo_G5.vi"() -> ("VIF_cluster"=w253:T22)  [unwired: 2 in, 1 out]
          }
          frame 6 {
            n143 = call "PM5000_VIF_demo_G6.vi"() -> ("VIF_cluster"=w254:T22)  [unwired: 2 in, 1 out]
          }
        }
      }
    }
    n144 = Unbundle By Name(w217) -> ("VL_VL"=w244:T23, "IL_IL"=w243:T24, "Frecuency"=w223:sgl)
    "?" <- w223
    n145 = Unbundle By Name(w243) -> ("I1"=w232:sgl, "I2"=w231:sgl, "I3"=w230:sgl, "Avg_Amps"=→"?":sgl)
    n146 = Unbundle By Name(w244) -> ("V1_V2"=w237:sgl, "V2_V3"=w236:sgl, "V3_V1"=w235:sgl, "Avg_VL_VL"=→"?":sgl)
    n147 = Bundle("I1"=w232, "I2"=w231, "I3"=w230) -> (→"Corriente L_L":cluster{"I1":sgl, "I2":sgl, "I3":sgl})  [unwired: 1 in]
    n148 = call "LimitAlarms.vi"("Value"=w239, "Parameter"=w240) -> ("Min"=w234:sgl, "Max"=w238:sgl)
    n149 = call "LimitAlarms.vi"("Value"=w227, "Parameter"=w226) -> ("Min"=w224:sgl, "Max"=w225:sgl)
    n150 = Bundle("Max"=w238, "V1_V2"=w237, "V2_V3"=w236, "V3_V1"=w235, "Min"=w234) -> (→"Voltaje L-L":T7)  [unwired: 1 in]
    n151 = Bundle("Max"=w225, "Frecuency"=w223, "Min"=w224) -> (→"Frecuencia":cluster{"Max":sgl, "Frecuency":sgl, "Min":sgl})  [unwired: 1 in]
    n152 = call "FGV_Stop_Local.vi"("Action"=enum16{"Read", "Write"}."Read") -> ("Error Out"=w219:errorcluster, "Var Out"=w221:bool)  [unwired: 9 in]
    n153 = call "Wait_Local.vi"("Wait time (msec)"=u32 1000 ("milliseconds to wait")) -> ()  [unwired: 5 in]
  }
  n154 = while {
    tunnel: [w257] -> w14
    tunnel: w3 -> [_]
    stop <- w255 stop-if-true
    # "Hora y Fecha"
    n155 = call "Fecha_HMI.vi"() -> ("fecha y hora"=→"fecha y hora":T2)  [unwired: 11 in]
    n156 = call "FGV_Stop_Local.vi"("Action"=enum16{"Read", "Write"}."Read") -> ("Error Out"=w257:errorcluster, "Var Out"=w255:bool)  [unwired: 9 in]
    n157 = call "Wait_Local.vi"("Wait time (msec)"=u32 1000 ("milliseconds to wait")) -> ()  [unwired: 5 in]
  }
  n158 = while {
    tunnel: [w260] -> w5
    tunnel: w3 -> [_]
    stop <- w261 stop-if-true
    # "Maneja Eventos de Usuario"
    n159 = event shown="[0] \"volver\": Value Change" {
      selector: _ -> [_ _]
      dyn-events: _ -> [_ _]
      timeout: _ -> [_ _]
      tunnel: [TRUE _] -> w261
      event Value Change {
        n160 = event-data() -> ()  [unwired: 1 in, 6 out]
        n161 = disable-structure shown="Disabled" {
          frame Disabled {
            # "Permite volver a la ventana HMI\nque se cerró antes"
            n162 = vi-ref "HMI_main.vi"() -> (w266:refnum<vi>)
            n163 = property class="VI"(reference=w266) -> (error out=w264:errorcluster, "Path"=w265:path)  [unwired: 1 in, 1 out]
            n164 = Open VI Reference(type specifier VI Refnum (for type only)="type specifier VI Refnum (for type only) 2", vi path=w265, options=128, error in (no error)=w264) -> (vi reference=w268:refnum<vi>, error out=w272:errorcluster)  [unwired: 2 in]
            n165 = call-by-ref "Start Asynchronous Call"(reference=w268, error in=w272) -> (reference out=w271:refnum<vi>, error out=w270:errorcluster)  [unwired: 12 in]
            n166 = Close Reference(reference=w271, error in (no error)=w270) -> ()  [unwired: 1 out]
          }
          frame Enabled {
          }
        }
      }
      event Menu Selection (User) {
        n167 = event-data() -> ()  [unwired: 1 in, 1 out]
        n168 = call "Display Message to User"() -> ()  [unwired: 10 in, 2 out]
      }
    }
    n169 = call "FGV_Stop_Local.vi"("Action"=enum16{"Read", "Write"}."Write", "Var In"=w261) -> ("Error Out"=w260:errorcluster)  [unwired: 8 in, 1 out]
  }
  n170 = Merge Errors(w5, w14, w13, w12, w11, w10, w9, w8, w6) -> (w7:errorcluster)
  n171 = call "Enqueue Error.vi"("error in"=w7) -> ("error out"=w4:errorcluster)  [unwired: 9 in, 1 out]
  n172 = flat-sequence {
    tunnel: w4 -> [_]
    frame #0 {
      n173 = control-ref of="This VI"() -> (w277:refnum<vi>)
      n174 = invoke class="VI" method="FP.Close"(reference=w277) -> (reference out=w274:refnum<vi>, error out=w273:errorcluster)  [unwired: 2 in, 1 out]
      n175 = Close Reference(reference=w274, error in (no error)=w273) -> ()  [unwired: 1 out]
      n176 = call "FGV_Stop_Local.vi"("Action"=enum16{"Read", "Write"}."Write", "Var In"=FALSE) -> ()  [unwired: 8 in, 2 out]
    }
  }
